vi "PromptForAttributes.vi"(9 "Attributes In":string[][](array[string]), 10 "Mouse Coords":T1, 11 "New Node Name":string) -> (2 "Canceled":bool, 3 "Attributes":string[][](array[string]))   [LabVIEW 2017]
uses:
  <vilib>/Utility/miscctls.llb/LVPoint32TypeDef.ctl
  <vilib>/Utility/Data Type/NI_Data Type.lvlib
panel:
  out "Array":variant[](array[variant])
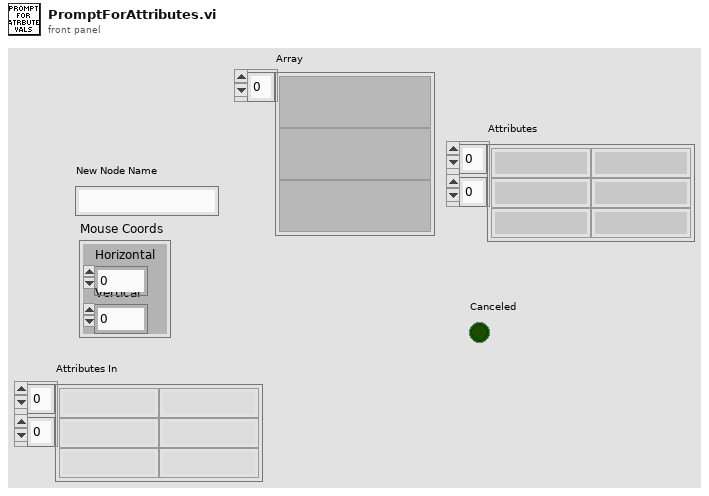
[diagram p1: front panel]
types:
  T1 = typedef "LVPoint32TypeDef.ctl" = cluster{"Horizontal":i32, "Vertical":i32}
  T2 = cluster{"Horizontal":i32, "Vertical":i32, "Horizontal":i32, "Vertical":i32}
  T3 = typedef "NI_Data Type.lvlib/Data Type.ctl" = enum8{"Invalid Type", "Void", "I8", "I16", "I32", "I64", "U8", "U16", "U32", "U64", "Single Float", "Double Float", "Extended Float", "Single Complex", "Double Complex", "Extended Complex", "Enum U8", "Enum U16", "Enum U32", "Enum U64", "Single Float With Unit", "Double Float With Unit", "Extended Float With Unit", "Single Complex with Unit", "Double Complex with Unit", "Extended Complex with Unit", "Boolean", "String", "Path", "Picture", "Tag", "Array", "Cluster", "Variant", "LV Variant", "Waveform", "Timestamp", "Digital Waveform", "Digital Data", "ExpressData", "Refnum", "External Data", "VI", "Poly VI", "LabVIEW Class Instance", "Fixed Point"}
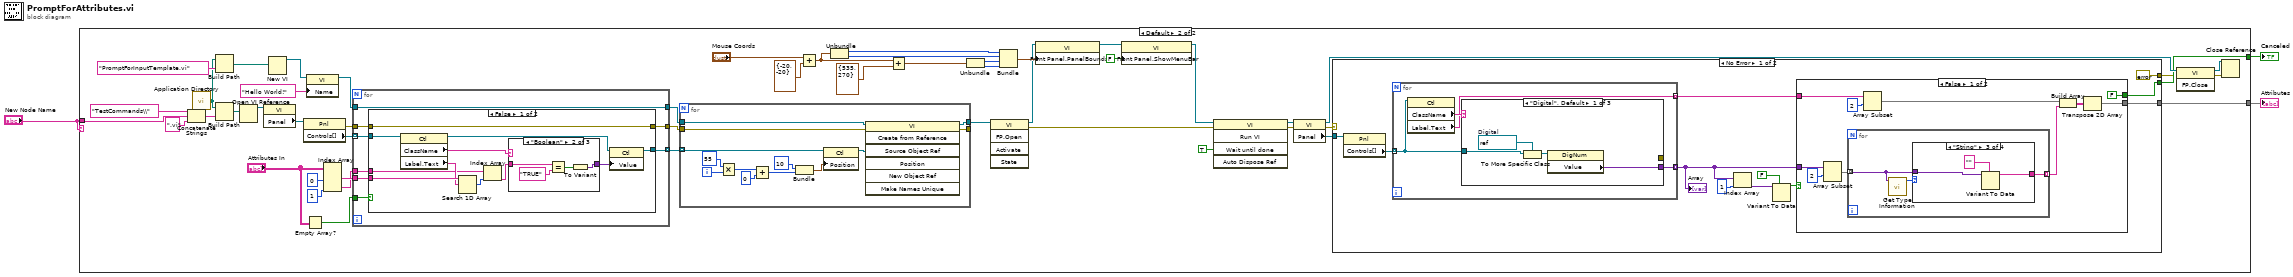
[diagram p0: block diagram]
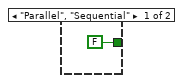
[diagram p2: hidden frame]
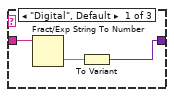
[diagram p3: hidden frame]
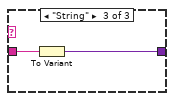
[diagram p4: hidden frame]
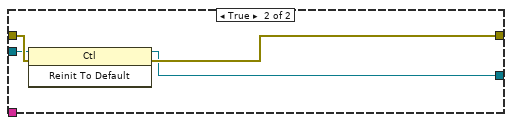
[diagram p5: hidden frame]
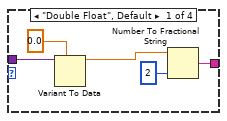
[diagram p6: hidden frame]
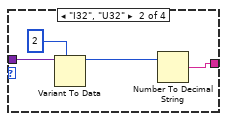
[diagram p7: hidden frame]
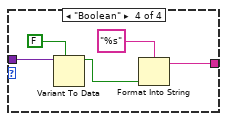
[diagram p8: hidden frame]
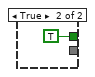
[diagram p9: hidden frame]
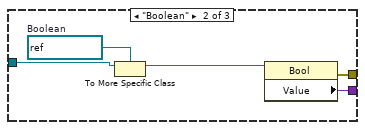
[diagram p10: hidden frame]
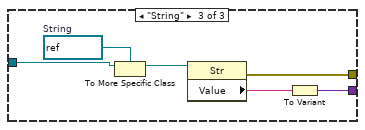
[diagram p11: hidden frame]
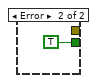
[diagram p12: hidden frame]
diagram:
  n1 = case shown="Default" "New Node Name" {
    tunnel: "New Node Name" -> [_ w44]
    tunnel: [FALSE ("Canceled") w37] -> w2
    tunnel: [_ w36] -> w1
    frame "Parallel", "Sequential" {
    }
    frame Default {
      n2 = Concatenate Strings("TestCommands\\" ("string"), w44, ".vi" ("string")) -> (w41:string)
      n3 = call <vilib>:"Application Directory.vi"() -> ("Application Directory"=w40:path)
      n4 = Build Path(base path=w40, name or relative path="PromptForInputTemplate.vi") -> (appended path=w45:path)
      n5 = Build Path(base path=w40, name or relative path=w41) -> (appended path=w39:path)
      n6 = Open VI Reference(vi path=w39) -> (vi reference=w21:refnum<vi>)  [unwired: 5 in, 1 out]
      n7 = property class="VI"(reference=w21) -> ("Panel"=w55:refnum<vi>)  [unwired: 1 in, 2 out]
      n8 = New VI(10:w45) -> (3:w50:refnum<vi>)  [unwired: 6 in, 1 out]
      n9 = property class="Pnl"(reference=w55) -> (error out=w13:errorcluster, "Controls[]"=w16:refnum<vi>[])  [unwired: 1 in, 1 out]
      n10 = property class="VI"(reference=w50, "Name"="Hello World!" ("VI Name")) -> (reference out=w11:refnum<vi>)  [unwired: 1 in, 1 out]
      n11 = Empty Array?(array="Attributes In") -> (empty?=w5:bool)
      n12 = Index Array(array="Attributes In", index (col) #1=0 ("disabled index (col)"), index (col) #2=1 ("index (col)")) -> (element #1=w9:string[], element #2=w7:string[])  [unwired: 2 in]
      n13 = for {
        tunnel: w16 -> [w61] mode=indexing
        tunnel: [w62] -> w15 mode=indexing
        tunnel: [w56] -> w14
        tunnel: w13 -> [w57]
        tunnel: [w63] -> w12
        tunnel: w11 -> [w63]
        tunnel: w9 -> [w60]
        tunnel: w7 -> [w59]
        tunnel: w5 -> [w58]
        n14 = case shown="False" w58 {
          tunnel: [w65 w85] -> w62
          tunnel: w61 -> [w74 w84]
          tunnel: w60 -> [w72 _]
          tunnel: w59 -> [w70 _]
          tunnel: w57 -> [w66 w87]
          tunnel: [w66 w86] -> w56
          frame False {
            n15 = property class="Ctl"(reference=w74) -> (reference out=w64:refnum<vi>, "ClassName"=w73:string, "Label.Text"=w71:string)  [unwired: 1 in, 1 out]
            n16 = Search 1D Array(1D array=w72, element=w71) -> (index of element=w69:i32)  [unwired: 1 in]
            n17 = Index Array(array=w70, index=w69) -> (element=w68:string)
            n18 = case shown="\"Boolean\"" w73 {
              tunnel: w68 -> [w77 w81 w83]
              tunnel: [w75 w78 w82] -> w67
              frame "Digital", Default {
                n19 = Fract/Exp String To Number(string=w77) -> (number=w76:dbl)  [unwired: 3 in, 1 out]
                n20 = To Variant(anything=w76) -> (Variant=w75:variant)
              }
              frame "Boolean" {
                n21 = Equal?(x=w81, y="TRUE") -> (x = y?=w79:bool)
                n22 = To Variant(anything=w79) -> (Variant=w78:variant)
              }
              frame "String" {
                n23 = To Variant(anything=w83) -> (Variant=w82:variant)
              }
            }
            n24 = property class="Ctl"(reference=w64, "Value"=w67) -> (reference out=w65:refnum<vi>)  [unwired: 1 in, 1 out]
          }
          frame True {
            n25 = invoke class="Ctl" method="Reinit To Default"(reference=w84, error in=w87) -> (reference out=w85:refnum<vi>, error out=w86:errorcluster)  [unwired: 1 in, 1 out]
          }
        }
      }
      n26 = for {
        tunnel: w12 -> [w162]
        tunnel: w14 -> [w161]
        tunnel: w15 -> [w150] mode=indexing
        tunnel: [w160] -> w17
        tunnel: [w159] -> _
        i -> [w158]
        n27 = Multiply(x=55, y=w158) -> (x*y=w156:i32)
        n28 = Add(x=w156, y=0) -> (x+y=w153:i32)
        n29 = Bundle("y"=10, w153) -> (w151:cluster{"y":i32, i32})  [unwired: 1 in]
        n30 = property class="Ctl"(reference=w150, "Position"=w151) -> (reference out=w154:refnum<vi>)  [unwired: 1 in, 1 out]
        n31 = invoke class="VI" method="Create from Reference"(reference=w162, error in=w161, "Source Object Ref"=w154) -> (reference out=w160:refnum<vi>, error out=w159:errorcluster)  [unwired: 4 in, 5 out]
      }
      n32 = Add(x="Mouse Coords", y=T1 {"Horizontal"=-20, "Vertical"=-20}) -> (x+y=w23:T1)
      n33 = Unbundle(w23) -> ("Horizontal"=w30:i32, "Vertical"=w29:i32)
      n34 = Add(x=w23, y=cluster{"Left":i16, "Top":i16} {"Left"=535, "Top"=270} ("Front Panel Window:Panel Bounds")) -> (x+y=w32:T1)
      n35 = Unbundle(w32) -> ("Horizontal"=w28:i32, "Vertical"=w27:i32)
      n36 = invoke class="VI" method="FP.Open"(reference=w17) -> (reference out=w20:refnum<vi>, error out=w49:errorcluster)  [unwired: 4 in, 3 out]
      n37 = Bundle("Horizontal"=w30, "Vertical"=w29, "Horizontal"=w28, "Vertical"=w27) -> (w26:T2)  [unwired: 1 in]
      n38 = property class="VI"(reference=w20, "Front Panel.PanelBounds"=w26) -> (reference out=w19:refnum<vi>)  [unwired: 1 in, 1 out]
      n39 = property class="VI"(reference=w19, "Front Panel.ShowMenuBar"=FALSE ("Front Panel Window:Show Menu Bar")) -> (reference out=w18:refnum<vi>)  [unwired: 1 in, 1 out]
      n40 = invoke class="VI" method="Run VI"(reference=w18, error in=w49, "Wait until done"=TRUE ("Wait Until Done")) -> (reference out=w51:refnum<vi>, error out=w52:errorcluster)  [unwired: 2 in, 3 out]
      n41 = property class="VI"(reference=w51, error in=w52) -> (reference out=w54:refnum<vi>, error out=w38:errorcluster, "Panel"=w53:refnum<vi>)
      n42 = case shown="No Error" w38 {
        tunnel: w53 -> [w97 _]
        tunnel: [w93 TRUE ("Canceled")] -> w37
        tunnel: [w90 _] -> w36
        tunnel: [errorcluster {"status"=FALSE, "code"=0, "source"=""} ("error constant") _] -> w33
        frame No Error {
          n43 = property class="Pnl"(reference=w97) -> ("Controls[]"=w98:refnum<vi>[])  [unwired: 1 in, 2 out]
          n44 = for {
            tunnel: w98 -> [w133] mode=indexing
            tunnel: [w131] -> w92 mode=indexing
            tunnel: [w130] -> w89 mode=indexing
            n45 = property class="Ctl"(reference=w133) -> ("ClassName"=w132:string, "Label.Text"=w130:string)  [unwired: 1 in, 2 out]
            n46 = case shown="\"Digital\", Default" w132 {
              tunnel: [_ w140 w146] -> _
              tunnel: w133 -> [w135 w139 w145]
              tunnel: [w134 w138 w143] -> w131
              frame "Digital", Default {
                w137 = refnum<vi> refnum  # Digital
                n47 = To More Specific Class(target class=w137, reference=w135) -> (specific class reference=w136:refnum<vi>)  [unwired: 1 in, 1 out]
                n48 = property class="DigNum"(reference=w136) -> ("Value"=w134:variant)  [unwired: 1 in, 2 out]
              }
              frame "Boolean" {
                w142 = refnum<vi> refnum  # Boolean
                n49 = To More Specific Class(target class=w142, reference=w139) -> (specific class reference=w141:refnum<vi>)  [unwired: 1 in, 1 out]
                n50 = property class="Bool"(reference=w141) -> (error out=w140:errorcluster, "Value"=w138:variant)  [unwired: 1 in, 1 out]
              }
              frame "String" {
                w148 = refnum<vi> refnum  # String
                n51 = To More Specific Class(target class=w148, reference=w145) -> (specific class reference=w147:refnum<vi>)  [unwired: 1 in, 1 out]
                n52 = property class="Str"(reference=w147) -> (error out=w146:errorcluster, "Value"=w144:string)  [unwired: 1 in, 1 out]
                n53 = To Variant(anything=w144) -> (Variant=w143:variant)
              }
            }
          }
          "Array" <- w92
          n54 = Index Array(array=w92, index=1) -> (element=w96:variant)
          n55 = Variant To Data(type=FALSE, Variant=w96) -> (data=w94:bool)  [unwired: 1 in, 1 out]
          n56 = case shown="False" w94 {
            tunnel: [FALSE ("Wait Until Done") TRUE ("Wait Until Done")] -> w93
            tunnel: w92 -> [w107 _]
            tunnel: [w99 _] -> w90
            tunnel: w89 -> [w102 _]
            frame False {
              n57 = Array Subset(array=w107, index=2) -> (w105:variant[])  [unwired: 1 in]
              n58 = for {
                tunnel: w105 -> [w110] mode=indexing
                tunnel: [w109] -> w104 mode=indexing
                n59 = call <vilib>:"Get Type Information.vi"("Variant"=w110) -> ("Type"=w111:T3)  [unwired: 6 in, 4 out]
                n60 = case shown="\"String\"" w111 {
                  tunnel: w110 -> [w114 w119 w123 w128]
                  tunnel: [w112 w118 w121 w126] -> w109
                  frame "Double Float", Default {
                    n61 = Variant To Data(type=0.0, Variant=w114) -> (data=w116:dbl)  [unwired: 1 in, 1 out]
                    n62 = Number To Fractional String(number=w116, precision (6)=i16 2) -> (F-format string=w112:string)  [unwired: 2 in]
                  }
                  frame "I32", "U32" {
                    n63 = Variant To Data(type=i16 2 ("precision (6)"), Variant=w119) -> (data=w120:i16)  [unwired: 1 in, 1 out]
                    n64 = Number To Decimal String(number=w120) -> (decimal integer string=w118:string)  [unwired: 1 in]
                  }
                  frame "String" {
                    n65 = Variant To Data(type="", Variant=w123) -> (data=w121:string)  [unwired: 1 in, 1 out]
                  }
                  frame "Boolean" {
                    n66 = Variant To Data(type=FALSE ("Wait Until Done"), Variant=w128) -> (data=w124:bool)  [unwired: 1 in, 1 out]
                    n67 = Format Into String(format string="%s", w124) -> (resulting string=w126:string)  [unwired: 2 in, 1 out]
                  }
                }
              }
              n68 = Array Subset(array=w102, index=2) -> (w101:string[])  [unwired: 1 in]
              n69 = Build Array(w101, w104) -> (w100:string[][])
              n70 = Transpose 2D Array(2D array=w100) -> (transposed array=w99:string[][])
            }
            frame True {
            }
          }
        }
        frame Error {
        }
      }
      n71 = invoke class="VI" method="FP.Close"(reference=w54, error in=w33) -> (reference out=w35:refnum<vi>, error out=w34:errorcluster)  [unwired: 1 in, 1 out]
      n72 = Close Reference(reference=w35, error in (no error)=w34) -> ()  [unwired: 1 out]
    }
  }
  "Attributes" <- w1
  "Canceled" <- w2
